vi "Listen and reply broadcast.ping.vi"(0 "service name":string="monitor", 1 "broker":string="dorian.t2", 2 "driplineinfolocation":path, 3 "error (in)":errorcluster) -> ()   [LabVIEW 2016]
uses:
  <vilib>/Distrio/LabbitMQ/Connection/Connection.lvclass
  <vilib>/Distrio/LabbitMQ/Queue/Queue.lvclass
  <vilib>/Distrio/LabbitMQ/Exchange/Exchange.lvclass
panel:
  in  "Stop Button":bool
  out "Listening to messages?":bool
  out "Execution:State":T1(ring)
  in  "recreate queue":bool
  in  "Tab Control":enum32{"AMQP Settings", "Logger"}(tab)
  out "binding keys":string[](array[string])
  out "error out":errorcluster
  out "error closing out":errorcluster
  out "Log":string
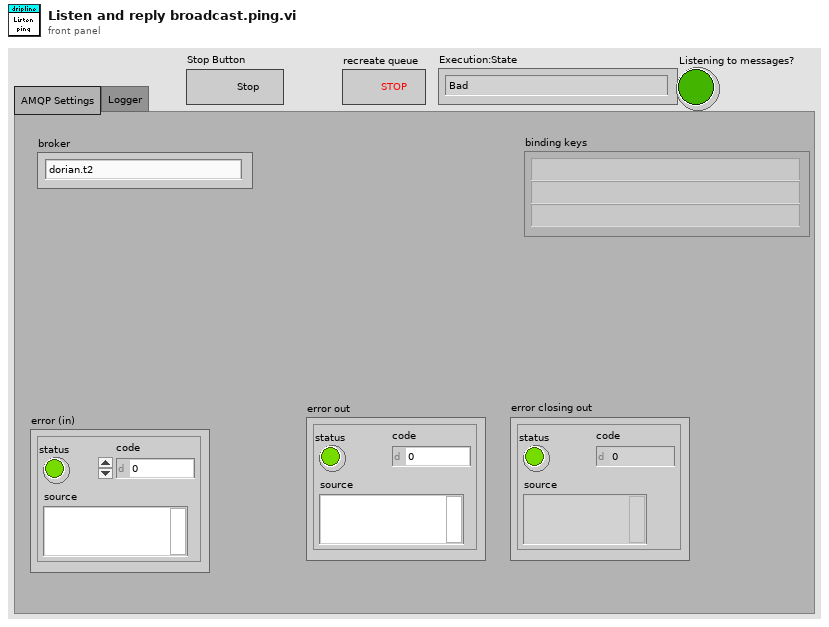
[diagram p1: front panel]
types:
  T1 = enum32{"Bad", "Idle", "Run top level", "Running"}
  T2 = cluster{"Exchange.lvclass":refnum<class "Exchange.lvclass">, "Queue out":refnum<class "Queue.lvclass">, "error out":errorcluster}
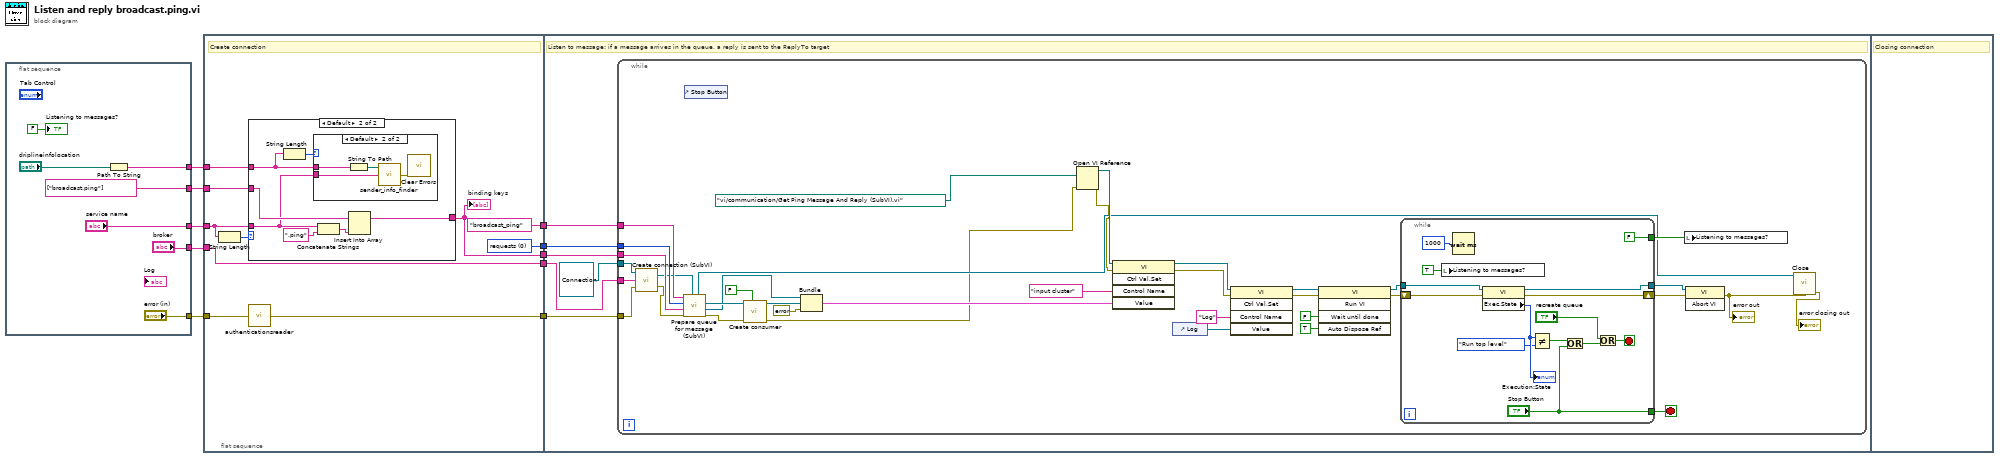
[diagram p0: block diagram]
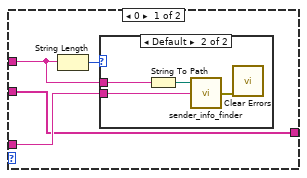
[diagram p2: hidden frame]
diagram:
  n1 = flat-sequence {
    tunnel: ["error (in)"] -> w10
    tunnel: ["broker"] -> w9
    tunnel: ["service name"] -> w8
    tunnel: [w12] -> w7
    tunnel: [string[] ["broadcast.ping"] ("broadcast.ping")] -> w6
    frame #0 {
      n2 = Path To String(path="driplineinfolocation") -> (string=w12:string)
      "Listening to messages?" <- FALSE ("Listening to messages?")
    }
  }
  n3 = flat-sequence {
    tunnel: [w20] -> w5
    tunnel: w9 -> [w21]
    tunnel: w10 -> [w27]
    tunnel: w8 -> [w25]
    tunnel: w7 -> [w26]
    tunnel: [w24] -> w4
    tunnel: w6 -> [w23]
    tunnel: [w21] -> w3
    tunnel: [w19] -> w2
    tunnel: ["broadcast_ping" ("queue name")] -> w1
    tunnel: w5 -> [w47]
    tunnel: w4 -> [w52]
    tunnel: w3 -> [w48]
    tunnel: w2 -> [w51]
    tunnel: w1 -> [w50]
    frame #0 {
      w19 = u16 0 items=["requests", "alerts"] ("exchange name")
      # "Create connection"
      n4 = String Length(string=w25) -> (length=w22:i32)
      n5 = case shown="Default" w22 {
        tunnel: w26 -> [w28 w41]
        tunnel: w25 -> [w31 w36]
        tunnel: [w30 w38] -> w24
        tunnel: w23 -> [w30 w37]
        frame 0 {
          n6 = String Length(string=w28) -> (length=w29:i32)
          n7 = case shown="Default" w29 {
            tunnel: w31 -> [_ w35]
            tunnel: w28 -> [_ w32]
            frame 0 {
            }
            frame Default {
              n8 = String To Path(string=w32) -> (path=w34:path)
              n9 = call "sender_info_finder.vi"("service name"=w35, "file (use dialog)"=w34) -> ("error (out)"=w33:errorcluster)  [unwired: 1 in]
              n10 = call <vilib>:"Clear Errors.vi"("error in (no error)"=w33) -> ()  [unwired: 5 in, 2 out]
            }
          }
        }
        frame Default {
          n11 = String Length(string=w41) -> (length=w42:i32)
          n12 = case shown="Default" w42 {
            tunnel: w36 -> [_ w46]
            tunnel: w41 -> [_ w43]
            frame 0 {
            }
            frame Default {
              n13 = String To Path(string=w43) -> (path=w45:path)
              n14 = call "sender_info_finder.vi"("service name"=w46, "file (use dialog)"=w45) -> ("error (out)"=w44:errorcluster)  [unwired: 1 in]
              n15 = call <vilib>:"Clear Errors.vi"("error in (no error)"=w44) -> ()  [unwired: 5 in, 2 out]
            }
          }
          n16 = Concatenate Strings(w36, ".ping" ("string")) -> (w39:string)
          n17 = Insert Into Array(array=w37, new element=w39) -> (w38:string[])  [unwired: 1 in]
        }
      }
      "binding keys" <- w24
      n18 = call "authenticationsreader.vi"("error (in)"=w27) -> ("error (out)"=w20:errorcluster)
    }
    frame #1 {
      # "Listen to message: if a message arrives in the queue, a reply is sent to the ReplyTo target"
      n19 = while {
        tunnel: w52 -> [w86]
        tunnel: w50 -> [w85]
        tunnel: w51 -> [w84]
        tunnel: refnum<class "Connection.lvclass"> refnum ("Connection in") -> [w63]
        tunnel: w48 -> [w62]
        tunnel: w47 -> [w59]
        stop <- w75 stop-if-true
        n20 = call "Create connection (SubVI).vi"("error in (no error)"=w59, "host name"=w62, "Connection in"=w63) -> ("error out"=w61:errorcluster, "Connection out"=w60:refnum<class "Connection.lvclass">)
        n21 = call "Prepare queue for message (SubVI).vi"("Connection in"=w60, "error in (no error)"=w61, "binding key"=w86, "exchange name"=w84, "queue \nname"=w85) -> ("error out"=w88:errorcluster, "Exchange.lvclass"=w81:refnum<class "Exchange.lvclass">, "Queue out"=w87:refnum<class "Queue.lvclass">, "Connection out"=w65:refnum<class "Connection.lvclass">)  [unwired: 1 out]
        n22 = control-ref of="Stop Button"() -> ()  [unwired: 1 out]
        n23 = call <vilib>:"Create consumer.vi"("noAck? (T)"=FALSE, "error in (no error)"=w88, "Queue in"=w87) -> ("error out"=w56:errorcluster, "Queue out"=w80:refnum<class "Queue.lvclass">)  [unwired: 7 in]
        n24 = Bundle("Exchange.lvclass"=w81, "Queue out"=w80, "error out"=errorcluster {"status"=FALSE, "code"=0, "source"=""}) -> (w74:T2)  [unwired: 1 in]
        n25 = Open VI Reference(vi path=path "vi/communication/Get Ping Message And Reply (SubVI).vi", error in (no error)=w56) -> (vi reference=w83:refnum<vi>, error out=w55:errorcluster)  [unwired: 4 in]
        n26 = invoke class="VI" method="Ctrl Val.Set"(reference=w83, error in=w55, "Control Name"="input cluster", "Value"=w74) -> (reference out=w68:refnum<vi>, error out=w67:errorcluster)  [unwired: 1 in, 3 out]
        n27 = control-ref of="Log"() -> (w69:refnum<vi>)
        n28 = invoke class="VI" method="Ctrl Val.Set"(reference=w68, error in=w67, "Control Name"="Log", "Value"=w69) -> (reference out=w72:refnum<vi>, error out=w54:errorcluster)  [unwired: 1 in, 3 out]
        n29 = invoke class="VI" method="Run VI"(reference=w72, error in=w54, "Wait until done"=FALSE ("Wait Until Done"), "Auto Dispose Ref"=TRUE ("Auto Dispose Reference")) -> (reference out=w77:refnum<vi>, error out=w53:errorcluster)  [unwired: 1 in, 3 out]
        n30 = while {
          tunnel: w77 -> [w101]
          tunnel: [w100] -> w73
          tunnel: [FALSE] -> w76
          shift-right: [w94] -> w66
          shift-left: w53 -> [w95]
          tunnel: ["Stop Button"] -> w75
          stop <- w92 stop-if-true
          n31 = local write "Listening to messages?"(TRUE ("broadcast.ping listener?")) -> ()
          n32 = Wait (ms)(milliseconds to wait=u32 1000) -> ()  [unwired: 1 out]
          n33 = property class="VI"(reference=w101, error in=w95) -> (reference out=w100:refnum<vi>, error out=w94:errorcluster, "Exec.State"=w99:T1)
          "Execution:State" <- w99
          n34 = Not Equal?(x=w99, y=T1."Run top level") -> (x != y?=w96:bool)
          n35 = Or(x=w96, y="Stop Button") -> (x .or. y?=w97:bool)
          n36 = Or(x="recreate queue", y=w97) -> (x .or. y?=w92:bool)
        }
        n37 = local write "Listening to messages?"(w76) -> ()
        n38 = invoke class="VI" method="Abort VI"(reference=w73, error in=w66) -> (error out=w64:errorcluster)  [unwired: 1 in, 2 out]
        "error out" <- w64
        n39 = call <vilib>:"Close.vi"("error in (no error)"=w64, "Connection in"=w65) -> ("error out"=→"error closing out":errorcluster)  [unwired: 8 in, 1 out]
      }
    }
    frame #2 {
      # "Closing connection"
    }
  }
